vi "FindRouteExample.vi"() -> ()   [LabVIEW 2009]
uses:
  PathTree/RouteTree.lvclass
  Waypoint/point.ctl
  Waypoint/Waypoint.lvclass
panel:
  out "BestTime":u32 caption="Time (ms)"
  out "Best Distance":dbl caption="Distance"
  in  "Best Solve":bool
  out "SmartTime":u32 caption="Time (ms)"
  out "Smart Distance":dbl caption="Distance"
  in  "Smart Solve":bool
  out "FastTime":u32 caption="Time (ms)"
  out "Fast Distance":dbl caption="Distance"
  in  "Fast Solve":bool
  in  "NumPoints":i32
  in  "NewPoints":bool
  in  "Exit":bool
  out "Paths":picture
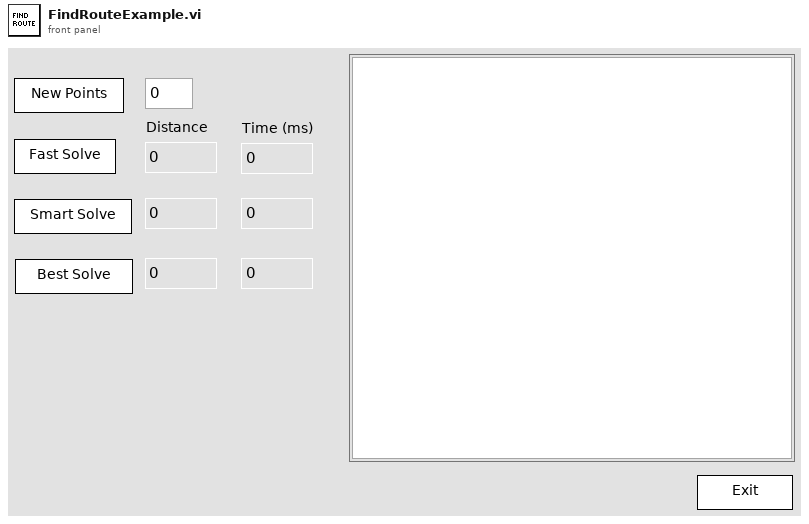
[diagram p1: front panel]
types:
  T1 = typedef "Waypoint.lvclass/point.ctl" = cluster{"X":dbl, "Y":dbl}
  T2 = cluster{"Width":u16, "Style":enum32{"Solid", "Dash", "Dot", "DashDot", "DashDotDot"}}
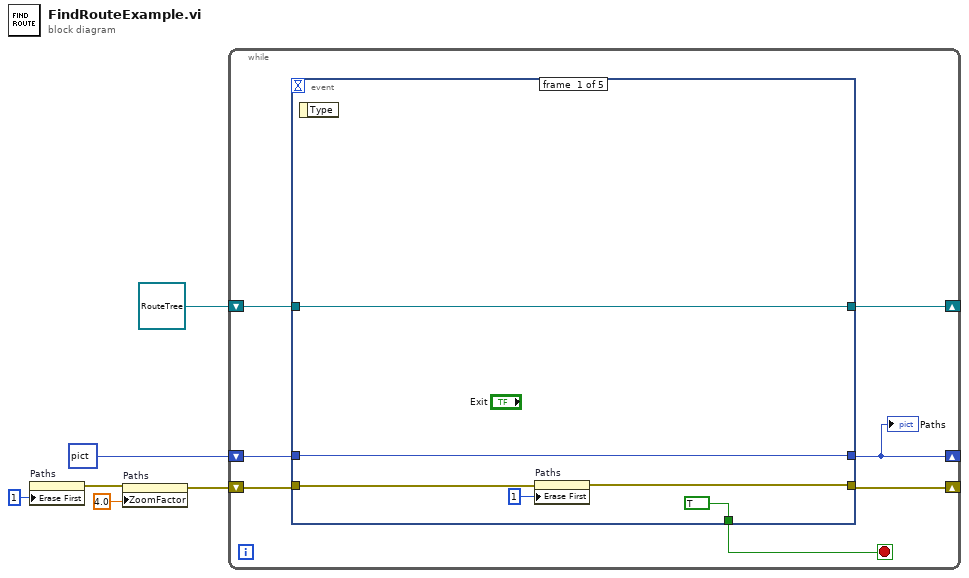
[diagram p0: block diagram]
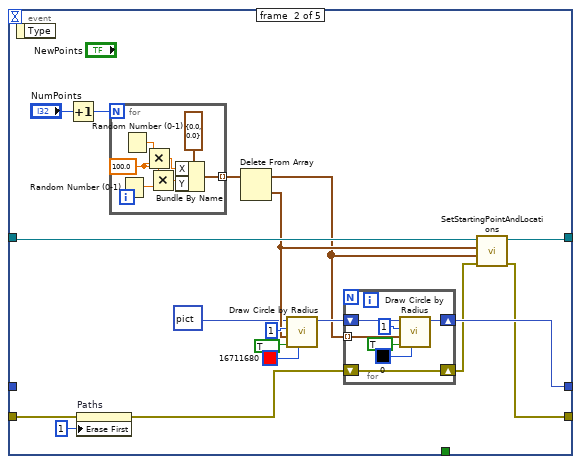
[diagram p2: hidden frame]
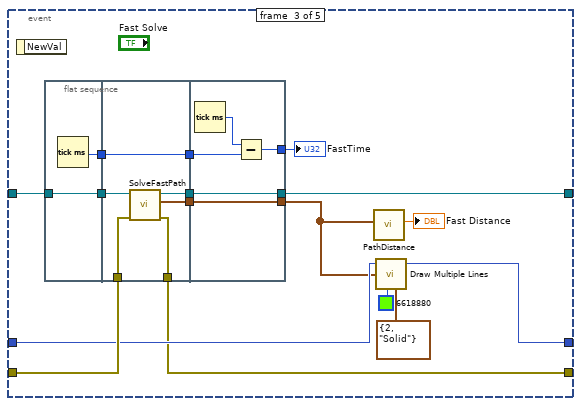
[diagram p3: hidden frame]
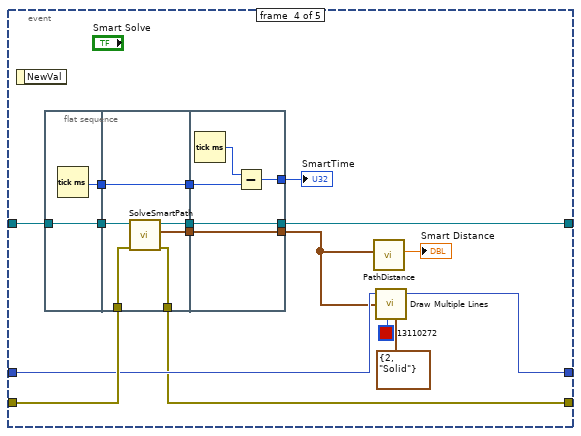
[diagram p4: hidden frame]
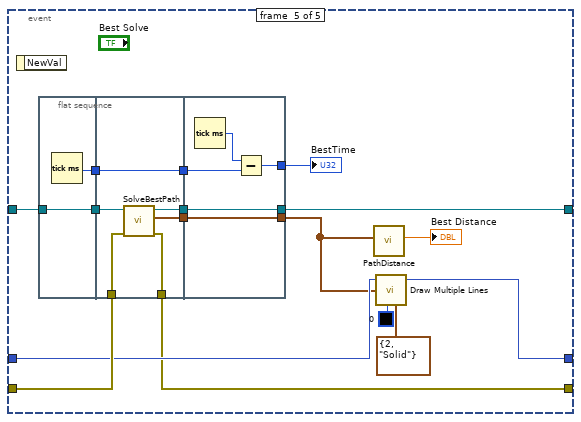
[diagram p5: hidden frame]
diagram:
  n1 = property on="Paths" class="Pict"("Erase First"=u8 1) -> (error out=w1:errorcluster)  [unwired: 2 in, 1 out]
  n2 = property on="Paths" class="Pict"(error in=w1, "ZoomFactor"=sgl 4.0 ("Zoom Factor")) -> (error out=w4:errorcluster)  [unwired: 1 in, 1 out]
  n3 = while {
    shift-right: [w7] -> _
    shift-left: picture data[5B] ("Paths") -> [w10]
    shift-right: [w8] -> _
    shift-left: w4 -> [w9]
    shift-right: [w12] -> _
    shift-left: refnum<class "RouteTree.lvclass"> refnum ("RouteTree.lvclass") -> [w13]
    stop <- w11 stop-if-true
    n4 = event shown="[3] \"Smart Solve\": Value Change" {
      selector: _ -> [_ _ _ _ _]
      dyn-events: _ -> [_ _ _ _ _]
      timeout: _ -> [_ _ _ _ _]
      tunnel: w13 -> [w19 w26 w67 w96 w125]
      tunnel: [w19 w25 w66 w95 w124] -> w12
      tunnel: [TRUE _ _ _ _] -> w11
      tunnel: w10 -> [w17 _ w64 w93 w122]
      tunnel: [w17 w27 w61 w90 w119] -> w7
      tunnel: w9 -> [w16 w29 w65 w94 w123]
      tunnel: [w14 w21 w60 w89 w118] -> w8
      event #0 {
        n5 = event-data() -> ()  [unwired: 1 in, 1 out]
        n6 = property on="Paths" class="Pict"(error in=w16, "Erase First"=u8 1) -> (error out=w14:errorcluster)  [unwired: 1 in, 1 out]
      }
      event #1 {
        n7 = event-data() -> ()  [unwired: 1 in, 1 out]
        n8 = Increment(x="NumPoints") -> (x+1=w37:i32)
        n9 = property on="Paths" class="Pict"(error in=w29, "Erase First"=u8 1) -> (error out=w28:errorcluster)  [unwired: 1 in, 1 out]
        n10 = for {
          N: w37 -> [_]
          tunnel: [w45] -> w35 mode=indexing
          w47 = 100.0 ("x")
          n11 = Random Number (0-1)() -> (number: 0 to 1=w49:dbl)
          n12 = Random Number (0-1)() -> (number: 0 to 1=w51:dbl)
          n13 = Multiply(x=w51, y=w47) -> (x*y=w50:dbl)
          n14 = Multiply(x=w47, y=w49) -> (x*y=w48:dbl)
          n15 = Bundle By Name(cluster=T1 {"X"=0.0, "Y"=0.0} ("point"), "X"=w50, "Y"=w48) -> (w45:T1)
        }
        n16 = Delete From Array(array=w35) -> (deleted portion=w24:T1, array with subset deleted=w23:T1[])  [unwired: 2 in]
        n17 = call <vilib>:"Draw Circle by Radius.vi"("color(black)"=u32 16711680, "fill?(F)"=TRUE, "pixel center"=w24, "radius"=i16 1, "picture"=picture data[5B]) -> ("new picture"=w31:picture)  [unwired: 6 in]
        n18 = for {
          shift-right: [w40] -> w27
          shift-left: w31 -> [w41]
          shift-right: [w39] -> w22
          shift-left: w28 -> [w39]
          tunnel: w23 -> [w38] mode=indexing
          n19 = call <vilib>:"Draw Circle by Radius.vi"("color(black)"=u32 0, "fill?(F)"=TRUE, "pixel center"=w38, "radius"=i16 1, "picture"=w41) -> ("new picture"=w40:picture)  [unwired: 6 in]
        }
        n20 = call "SetStartingPointAndLocations.vi"("error in (no error)"=w22, "locations"=w23, "point"=w24, "PathTree in"=w26) -> ("error out"=w21:errorcluster, "PathTree out"=w25:refnum<class "RouteTree.lvclass">)  [unwired: 6 in]
      }
      event #2 {
        n21 = event-data() -> ()  [unwired: 1 in, 1 out]
        n22 = flat-sequence {
          tunnel: w67 -> [w69]
          tunnel: [w69] -> w55
          tunnel: [w68] -> w54
          tunnel: w65 -> [w73]
          tunnel: [w72] -> w60
          tunnel: [w74] -> w57
          tunnel: [w71] -> w56
          tunnel: w55 -> [w75]
          tunnel: w54 -> [w70]
          tunnel: [w70] -> w53
          tunnel: [w79] -> w59
          tunnel: [w80] -> w66
          tunnel: w57 -> [w80]
          tunnel: w56 -> [w79]
          tunnel: w53 -> [w77]
          tunnel: [w76] -> w52
          frame #0 {
            n23 = Tick Count (ms)() -> (millisecond timer value=w68:u32)
          }
          frame #1 {
            n24 = call "SolveFastPath.vi"("error in (no error)"=w73, "RouteTree in"=w75) -> ("error out"=w72:errorcluster, "greedy Path"=w71:T1[], "RouteTree out"=w74:refnum<class "RouteTree.lvclass">)  [unwired: 7 in]
          }
          frame #2 {
            n25 = Tick Count (ms)() -> (millisecond timer value=w78:u32)
            n26 = Subtract(x=w78, y=w77) -> (x-y=w76:u32)
          }
        }
        n27 = call "PathDistance.vi"("path"=w59) -> ("distance"=→"Fast Distance":dbl)  [unwired: 10 in]
        n28 = call <vilib>:"Draw Multiple Lines.vi"("picture"=w64, "line endpoints"=w59, "color(black)"=u32 6618880, "pen"=T2 {"Width"=2, "Style"=enum."Solid"}) -> ("new picture"=w61:picture)  [unwired: 5 in]
        "FastTime" <- w52
      }
      event #3 {
        n29 = event-data() -> ()  [unwired: 1 in, 1 out]
        n30 = flat-sequence {
          tunnel: w96 -> [w98]
          tunnel: [w98] -> w85
          tunnel: [w97] -> w84
          tunnel: w94 -> [w102]
          tunnel: [w101] -> w89
          tunnel: [w103] -> w87
          tunnel: [w100] -> w86
          tunnel: w85 -> [w104]
          tunnel: w84 -> [w99]
          tunnel: [w99] -> w83
          tunnel: [w108] -> w88
          tunnel: [w109] -> w95
          tunnel: w87 -> [w109]
          tunnel: w86 -> [w108]
          tunnel: w83 -> [w106]
          tunnel: [w105] -> w82
          frame #0 {
            n31 = Tick Count (ms)() -> (millisecond timer value=w97:u32)
          }
          frame #1 {
            n32 = call "SolveSmartPath.vi"("error in (no error)"=w102, "RouteTree in"=w104) -> ("error out"=w101:errorcluster, "Best First Path"=w100:T1[], "RouteTree out"=w103:refnum<class "RouteTree.lvclass">)  [unwired: 6 in, 1 out]
          }
          frame #2 {
            n33 = Tick Count (ms)() -> (millisecond timer value=w107:u32)
            n34 = Subtract(x=w107, y=w106) -> (x-y=w105:u32)
          }
        }
        n35 = call "PathDistance.vi"("path"=w88) -> ("distance"=→"Smart Distance":dbl)  [unwired: 10 in]
        n36 = call <vilib>:"Draw Multiple Lines.vi"("picture"=w93, "line endpoints"=w88, "color(black)"=u32 13110272, "pen"=T2 {"Width"=2, "Style"=enum."Solid"}) -> ("new picture"=w90:picture)  [unwired: 5 in]
        "SmartTime" <- w82
      }
      event #4 {
        n37 = event-data() -> ()  [unwired: 1 in, 1 out]
        n38 = flat-sequence {
          tunnel: w125 -> [w127]
          tunnel: [w127] -> w114
          tunnel: [w126] -> w113
          tunnel: w123 -> [w131]
          tunnel: [w130] -> w118
          tunnel: [w132] -> w116
          tunnel: [w129] -> w115
          tunnel: w114 -> [w133]
          tunnel: w113 -> [w128]
          tunnel: [w128] -> w112
          tunnel: [w138] -> w117
          tunnel: [w134] -> w124
          tunnel: w116 -> [w134]
          tunnel: w115 -> [w138]
          tunnel: w112 -> [w136]
          tunnel: [w135] -> w111
          frame #0 {
            n39 = Tick Count (ms)() -> (millisecond timer value=w126:u32)
          }
          frame #1 {
            n40 = call "SolveBestPath.vi"("error in (no error)"=w131, "RouteTree in"=w133) -> ("error out"=w130:errorcluster, "Path"=w129:T1[], "RouteTree out"=w132:refnum<class "RouteTree.lvclass">)  [unwired: 6 in, 1 out]
          }
          frame #2 {
            n41 = Tick Count (ms)() -> (millisecond timer value=w137:u32)
            n42 = Subtract(x=w137, y=w136) -> (x-y=w135:u32)
          }
        }
        n43 = call "PathDistance.vi"("path"=w117) -> ("distance"=→"Best Distance":dbl)  [unwired: 10 in]
        n44 = call <vilib>:"Draw Multiple Lines.vi"("picture"=w122, "line endpoints"=w117, "color(black)"=u32 0, "pen"=T2 {"Width"=2, "Style"=enum."Solid"}) -> ("new picture"=w119:picture)  [unwired: 5 in]
        "BestTime" <- w111
      }
    }
    "Paths" <- w7
  }
